vi "Write Power Supply classes.vi"(10 "Power Supply classes":refnum<class "Power Supply.lvclass">[](array[class]), 11 "Measurements in":refnum<class "Measurement.lvclass">) -> (3 "Measurements out":refnum<class "Measurement.lvclass">)   [LabVIEW 2020, in "Measurement.lvclass"]
uses:
  Measurement.lvclass
  Instruments/Power Supply/Power Supply.lvclass
  Measurement.lvclass/Measurement.ctl
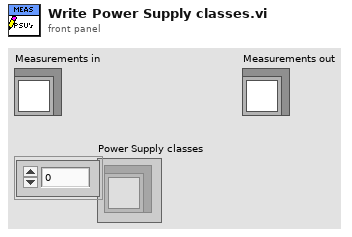
[diagram p1: front panel]
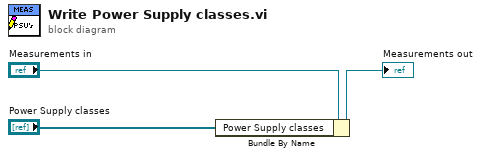
[diagram p0: block diagram]
diagram:
  n1 = Bundle By Name(cluster="Measurements in", "Power Supply classes"="Power Supply classes") -> (→"Measurements out":refnum<class "Measurement.lvclass">)
